vi "Initialize FGVs.vi"(8 "error in":errorcluster) -> (0 "error out":errorcluster)   [LabVIEW 2025]
uses:
  Types/XmlNodeDataActions.ctl
  Types/Section Map Action.ctl
  Types/TD NodeRef Map Action.ctl
  Types/CD NodeRef Map Action.ctl
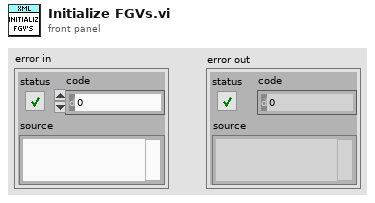
[diagram p1: front panel]
types:
  T1 = typedef "CD NodeRef Map Action.ctl" = enum16{"Init", "Add XMLNodeRef", "Update ParentName", "Delete XMLNodeRef", "Get All Keys", "Get", "skip"}
  T2 = typedef "TD NodeRef Map Action.ctl" = enum16{"Init", "Add XMLNodeRef", "Delete XMLNodeRef", "Add TDNodeRefs", "Delete TDNodeRefs", "Clear TDNodeRefs", "Add ChildXMLNodeRef", "Delete ChildXMLNodeRef", "Get All Keys", "Update ParentName", "Get", "skip"}
  T3 = typedef "Section Map Action.ctl" = enum16{"Delete Child Node", "Filter Valid Nodes", "Add Child Section", "Initialize"}
  T4 = typedef "XmlNodeDataActions.ctl" = enum16{"Init", "Add Channel", "Add Section", "Add Waveform", "Delete Channel", "Delete Section", "Delete Waveform", "Get Channels", "Get Sections", "Get Waveforms", "Skip", "Add Enum", "Get Enums", "Delete Enum"}
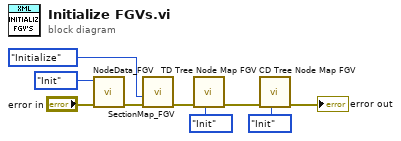
[diagram p0: block diagram]
diagram:
  n1 = call "NodeData_FGV.vi"("error in"="error in", "Action"=XmlNodeDataActions."Init") -> ("error out"=w8:errorcluster)  [unwired: 8 in, 1 out]
  n2 = call "SectionMap_FGV.vi"("error in"=w8, "Action"=Section_Map_Action."Initialize") -> ("error out"=w4:errorcluster)  [unwired: 8 in, 1 out]
  n3 = call "TD Tree Node Map FGV.vi"("Action"=TD_NodeRef_Map_Action."Init", "error in"=w4) -> ("error out"=w3:errorcluster)  [unwired: 4 in, 5 out]
  n4 = call "CD Tree Node Map FGV.vi"("Action"=CD_NodeRef_Map_Action."Init", "error in"=w3) -> ("error out"=→"error out":errorcluster)  [unwired: 5 in, 4 out]
